vi "itc ltc - aggregate.vi"(5 "aggregate every # sec":dbl=1.0, 7 "history length (min)":dbl=20.0, 11 "temperature boxes":T2={"LTC21 Address"="GPIB0::15::INSTR", "ITC503 Address"="GPIB0::24::INSTR", "ITC temperature"=299.2, "ITC set temperature"=295.0, "LTC temperature"=0.0, "heater"=0.0, "gas flow"=90.0, "P"=10.0, "D"=1.0, "I"=3.0, "ITC state"="X0A1C2S00H1L0\r", "nonzero temperature"=0.0, "Magn Field (T)"=0.0, "LakeShore340"="", "LS340 Adress"=0, "Sample Temperature Source"=enum."read T <- LakeShore 340", "Neocera sensor"=1}) -> (2 "temperature indicator panel":T1={"LTC T"=0.0, "ITC T"=299.2, "ITC Set T"=295.0, "LTC T slope, K/min"=-0.0, "heater i-average, V"=-0.0, "heater slope, V/min"=-0.0, "LTC T i-average, K"=0.0, "ITC T i-average, K"=0.0, "gas"=0.0} {"ITC Set T" format="%.3g"; "ITC T" format="%.3g"; "LTC T" format="%.3g"; "gas" format="%.3g"; "ITC T i-average, K" format="%#.5f"; "LTC T i-average, K" format="%#.5f"; "heater i-average, V" format="%.3g"; "heater slope, V/min" format="%#.5f"; "LTC T slope, K/min" format="%#.5f"})   [LabVIEW 2015]
uses:
  state.ctl
  Sample_Temperature_Source_Control.ctl
  temperature indicator.ctl
  aggregator - v - real - atomic.vi
  linear interpolation - real.vi
panel:
  in  "requested size":i32=1
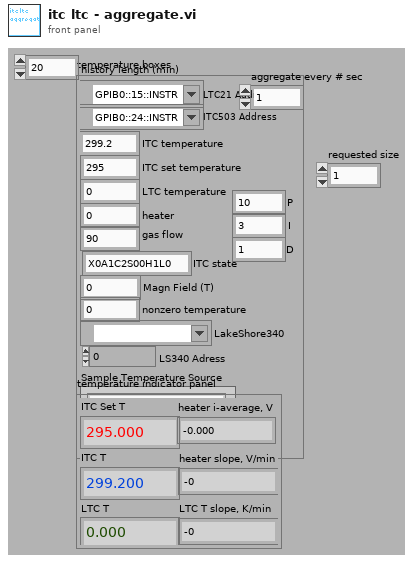
[diagram p1: front panel]
types:
  T1 = typedef "temperature indicator.ctl" = cluster{"LTC T":dbl, "ITC T":dbl, "ITC Set T":dbl, "LTC T slope, K/min":dbl, "heater i-average, V":dbl, "heater slope, V/min":dbl, "LTC T i-average, K":dbl, "ITC T i-average, K":dbl, "gas":dbl}
  T2 = typedef "state.ctl" = cluster{"LTC21 Address":refnum<visa-resource-name>, "ITC503 Address":refnum<visa-resource-name>, "ITC temperature":dbl, "ITC set temperature":dbl, "LTC temperature":dbl, "heater":dbl, "gas flow":dbl, "P":dbl, "D":dbl, "I":dbl, "ITC state":string, "nonzero temperature":dbl, "Magn Field (T)":dbl, "LakeShore340":refnum<visa-resource-name>, "LS340 Adress":i16, "Sample Temperature Source":T3, "Neocera sensor":i32}
  T3 = typedef "Sample_Temperature_Source_Control.ctl" = enum16{"read T <- LakeShore 340", "read T <- Neocera"}
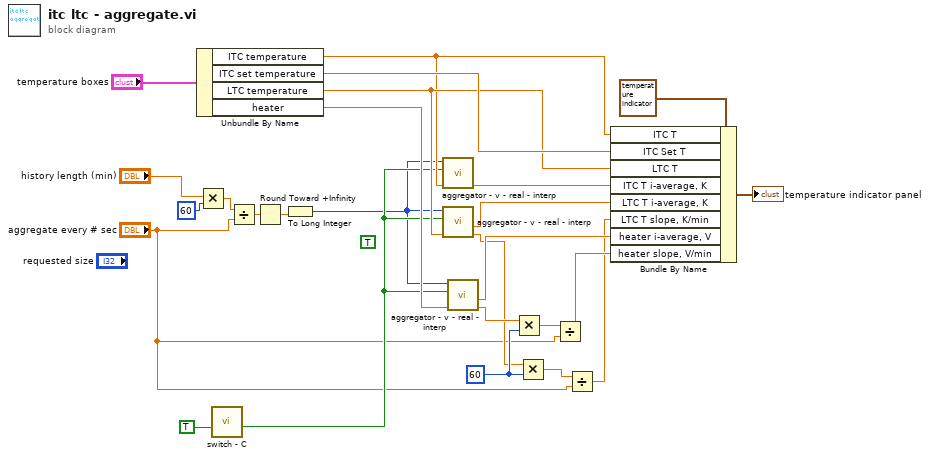
[diagram p0: block diagram]
diagram:
  (unwired) TRUE
  w8 = 60 ("y")
  n1 = Unbundle By Name("temperature boxes") -> ("ITC temperature"=w20:dbl, "ITC set temperature"=w24:dbl, "LTC temperature"=w21:dbl, "heater"=w16:dbl)
  n2 = Multiply(x="history length (min)", y=60) -> (x*y=w11:dbl)
  n3 = call "switch - C.vi"("switch"=TRUE) -> ("result"=w15:bool)  [unwired: 10 in]
  n4 = Divide(x=w11, y="aggregate every # sec") -> (x/y=w10:dbl)
  n5 = Round Toward +Infinity(x=w10) -> (ceil(x): smallest int >= x=w14:dbl)
  n6 = To Long Integer(number=w14) -> (32bit integer=w1:i32)
  n7 = call "aggregator - v - real - interp.vi"("number"=w20, "init?"=w15, "requested size"=w1) -> ("slope"=w19:dbl)  [unwired: 5 in, 3 out]
  n8 = call "aggregator - v - real - interp.vi"("number"=w21, "init?"=w15, "requested size"=w1) -> ("slope"=w7:dbl, "interp average"=w18:dbl)  [unwired: 5 in, 2 out]
  n9 = call "aggregator - v - real - interp.vi"("number"=w16, "init?"=w15, "requested size"=w1) -> ("slope"=w9:dbl, "interp average"=w17:dbl)  [unwired: 5 in, 2 out]
  n10 = Multiply(x=w9, y=w8) -> (x*y=w6:dbl)
  n11 = Multiply(x=w7, y=w8) -> (x*y=w3:dbl)
  n12 = Divide(x=w6, y="aggregate every # sec") -> (x/y=w5:dbl)
  n13 = Divide(x=w3, y="aggregate every # sec") -> (x/y=w4:dbl)
  n14 = Bundle By Name(cluster=T1 {"LTC T"=0.0, "ITC T"=0.0, "ITC Set T"=0.0, "LTC T slope, K/min"=0.0, "heater i-average, V"=0.0, "heater slope, V/min"=0.0, "LTC T i-average, K"=0.0, "ITC T i-average, K"=0.0, "gas"=0.0} ("temperature indicator panel 2"), "ITC T"=w20, "ITC Set T"=w24, "LTC T"=w21, "ITC T i-average, K"=w19, "LTC T i-average, K"=w18, "LTC T slope, K/min"=w4, "heater i-average, V"=w17, "heater slope, V/min"=w5) -> (→"temperature indicator panel":T1)
